vi "ma-resample unevenly sampled input (spline).vi"(0 "X-array in":dbl[](array[numeric]) format="%.2p", 5 "Y-array in":dbl[](array[numeric]) format="%.2p", 7 "dt":dbl=1.0 format="%.2p", 9 "t0":dbl format="%.2p", 11 "error in":errorcluster) -> (4 "X-array out":dbl[](array[numeric]) format="%.2p", 6 "Y-array out":dbl[](array[numeric]) format="%.2p", 8 "evenly sampled waveform out":waveform(dbl), 10 "used t0":dbl format="%.2p", 14 "t0 adjusted warning":bool, 15 "error out":errorcluster)   [LabVIEW 2020, in "NI_MAPro.lvlib"]
doc: "This VI re-samples an unevenly sampled input signal to an evenly sampled waveform according to specified t0 and dt. If the specified t0 value is less than the first value of input X-array (that is the timestamp of the first input sample), then the VI will coerce t0 to the first valid value (greater than X(0)) that also fulfill the relation:\n\nT0_adjusted - t0_in = n * dt_in\n\nThis guarranty that any later comparison of waveforms will be correct with repsect to absolute time."
uses:
  NI_MAPro.lvlib
  NI_AALPro.lvlib
  NI_AALBase.lvlib
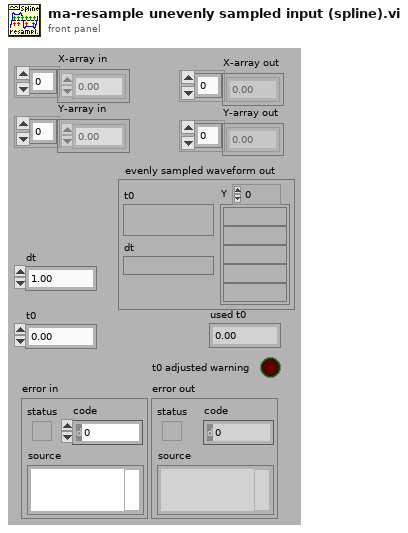
[diagram p1: front panel]
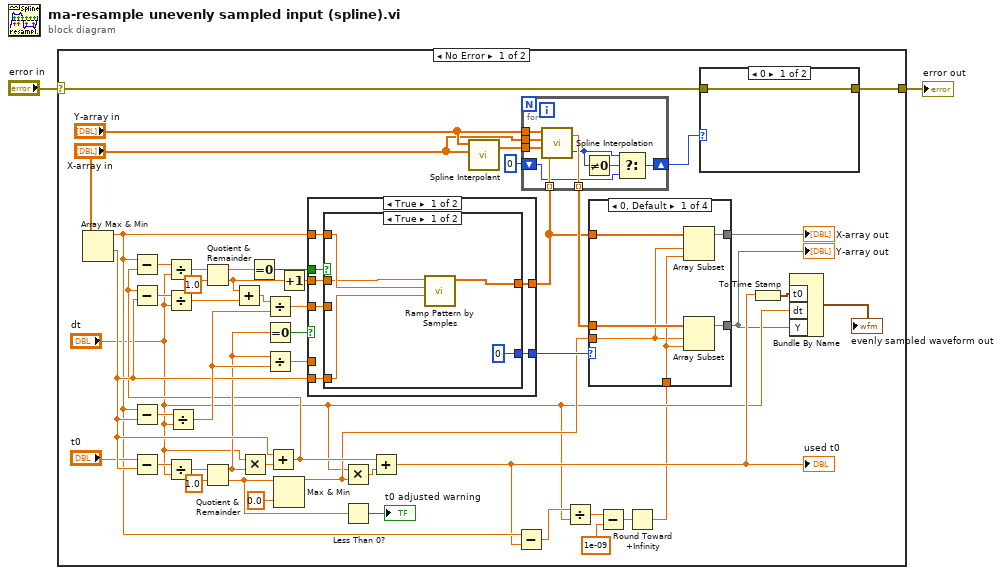
[diagram p0: block diagram]
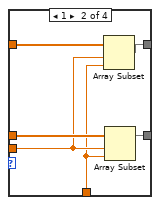
[diagram p2: hidden frame]
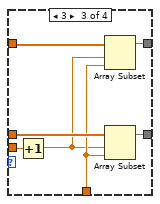
[diagram p3: hidden frame]
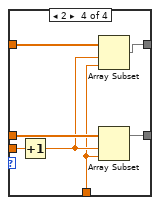
[diagram p4: hidden frame]
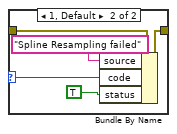
[diagram p5: hidden frame]
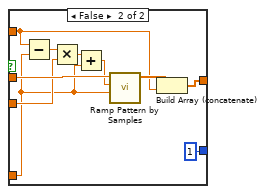
[diagram p6: hidden frame]
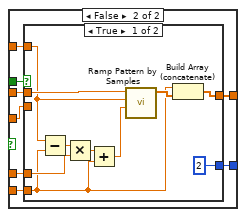
[diagram p7: hidden frame]
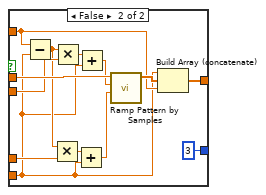
[diagram p8: hidden frame]
diagram:
  n1 = case shown="No Error" "error in" {
    selector: "error in" -> [w24 w147]
    tunnel: [w25 w147] -> w1
    frame No Error {
      n2 = Array Max & Min(array="X-array in") -> (max value=w17:dbl, min value=w31:dbl)  [unwired: 2 out]
      n3 = Subtract(x=w17, y=w31) -> (x-y=w41:dbl)
      n4 = Subtract(x="t0", y=w31) -> (x-y=w33:dbl)
      n5 = Divide(x=w33, y="dt") -> (x/y=w35:dbl)
      n6 = Divide(x=w41, y="dt") -> (x/y=w39:dbl)
      n7 = Quotient & Remainder(x=w35, y=1.0) -> (x-y*floor(x/y)=w30:dbl, floor(x/y)=w23:dbl)
      n8 = Multiply(x="dt", y=w30) -> (x*y=w32:dbl)
      n9 = Equal To 0?(x=w30) -> (x = 0?=w46:bool)
      n10 = Divide(x=w30, y=w39) -> (x/y=w44:dbl)
      n11 = Add(x=w31, y=w32) -> (x+y=w27:dbl)
      n12 = Subtract(x=w17, y=w27) -> (x-y=w50:dbl)
      n13 = Subtract(x=w27, y=w31) -> (x-y=w51:dbl)
      n14 = Divide(x=w50, y="dt") -> (x/y=w40:dbl)
      n15 = Divide(x=w51, y="dt") -> (x/y=w36:dbl)
      n16 = Quotient & Remainder(x=w40, y=1.0) -> (x-y*floor(x/y)=w48:dbl, floor(x/y)=w38:dbl)
      n17 = Add(x=w38, y=w36) -> (x+y=w37:dbl)
      n18 = Equal To 0?(x=w48) -> (x = 0?=w47:bool)
      n19 = Divide(x=w37, y=w39) -> (x/y=w45:dbl)
      n20 = Max & Min(x=w23, y=0.0) -> (max(x,y)=w20:dbl)  [unwired: 1 out]
      n21 = Increment(x=w38) -> (x+1=w42:dbl)
      n22 = case shown="True" w46 {
        tunnel: w47 -> [w91 w114]
        tunnel: w31 -> [w90 w113]
        tunnel: w17 -> [w89 w112]
        tunnel: [w88 w111] -> w18
        tunnel: w42 -> [w87 w110]
        tunnel: w45 -> [w86 w109]
        tunnel: w44 -> [_ w108]
        tunnel: [w85 w107] -> w21
        frame True {
          n23 = case shown="True" w91 {
            tunnel: w90 -> [w96 w98]
            tunnel: w89 -> [w95 w103]
            tunnel: [w94 w105] -> w88
            tunnel: w87 -> [w93 w106]
            tunnel: w86 -> [_ w101]
            tunnel: [0 1] -> w85
            frame True {
              n24 = call "Ramp Pattern by Samples.vi"("start"=w96, "end"=w95, "samples"=w93) -> ("Ramp Pattern"=w94:dbl[])  [unwired: 7 in, 1 out]
            }
            frame False {
              n25 = Subtract(x=w103, y=w98) -> (x-y=w102:dbl)
              n26 = Multiply(x=w102, y=w101) -> (x*y=w99:dbl)
              n27 = Add(x=w99, y=w98) -> (x+y=w100:dbl)
              n28 = call "Ramp Pattern by Samples.vi"("start"=w98, "end"=w100, "samples"=w106) -> ("Ramp Pattern"=w104:dbl[])  [unwired: 7 in, 1 out]
              n29 = Build Array (concatenate)(w104, w103) -> (w105:dbl[])
            }
          }
        }
        frame False {
          n30 = case shown="True" w114 {
            tunnel: w113 -> [w116 w127]
            tunnel: w112 -> [w121 w134]
            tunnel: [w118 w136] -> w111
            tunnel: w110 -> [w124 w137]
            tunnel: w109 -> [_ w133]
            tunnel: w108 -> [w120 w129]
            tunnel: [2 3] -> w107
            frame True {
              n31 = Subtract(x=w121, y=w116) -> (x-y=w123:dbl)
              n32 = Multiply(x=w123, y=w120) -> (x*y=w122:dbl)
              n33 = Add(x=w122, y=w116) -> (x+y=w119:dbl)
              n34 = call "Ramp Pattern by Samples.vi"("start"=w119, "end"=w121, "samples"=w124) -> ("Ramp Pattern"=w117:dbl[])  [unwired: 7 in, 1 out]
              n35 = Build Array (concatenate)(w116, w117) -> (w118:dbl[])
            }
            frame False {
              n36 = Subtract(x=w134, y=w127) -> (x-y=w128:dbl)
              n37 = Multiply(x=w128, y=w129) -> (x*y=w130:dbl)
              n38 = Multiply(x=w128, y=w133) -> (x*y=w131:dbl)
              n39 = Add(x=w130, y=w127) -> (x+y=w126:dbl)
              n40 = Add(x=w131, y=w127) -> (x+y=w132:dbl)
              n41 = call "Ramp Pattern by Samples.vi"("start"=w126, "end"=w132, "samples"=w137) -> ("Ramp Pattern"=w135:dbl[])  [unwired: 7 in, 1 out]
              n42 = Build Array (concatenate)(w127, w135, w134) -> (w136:dbl[])
            }
          }
        }
      }
      n43 = Multiply(x="dt", y=w20) -> (x*y=w29:dbl)
      n44 = Less Than 0?(x=w23) -> (x < 0?=→"t0 adjusted warning":bool)
      n45 = Add(x=w27, y=w29) -> (x+y=w16:dbl)
      "used t0" <- w16
      n46 = call "Spline Interpolant.vi"("X"="X-array in", "Y"="Y-array in") -> ("Interpolant"=w52:dbl[])  [unwired: 2 in, 1 out]
      n47 = Subtract(x=w17, y=w16) -> (x-y=w15:dbl)
      n48 = for {
        tunnel: w52 -> [w146]
        tunnel: "Y-array in" -> [w145]
        tunnel: w18 -> [w144] mode=indexing
        tunnel: [w143] -> w19 mode=indexing
        tunnel: "X-array in" -> [w140]
        shift-right: [w138] -> w4
        shift-left: 0 -> [w139]
        n49 = call "Spline Interpolation.vi"("x value"=w144, "Interpolant"=w146, "X"=w140, "Y"=w145) -> ("error"=w141:i32, "interpolation value"=w143:dbl)
        n50 = Not Equal To 0?(x=w141) -> (x != 0?=w142:bool)
        n51 = Select(t=w141, s=w142, f=w139) -> (s? t:f=w138:i32)
      }
      n52 = Divide(x=w15, y="dt") -> (x/y=w13:dbl)
      n53 = Subtract(x=w13, y=1e-09) -> (x-y=w11:dbl)
      n54 = Round Toward +Infinity(x=w11) -> (ceil(x): smallest int >= x=w10:dbl)
      n55 = case shown="0, Default" w21 {
        tunnel: w19 -> [w56 w63 w68 w77]
        tunnel: [w57 w64 w71 w78] -> w9
        tunnel: w18 -> [w55 w61 w70 w74]
        tunnel: [w58 w62 w69 w75] -> w8
        tunnel: w20 -> [w53 w60 w67 w73]
        tunnel: w10 -> [w54 w59 w66 w72]
        frame 0, Default {
          n56 = Array Subset(array=w55, index=w53, length=w54) -> (w58:dbl[])
          n57 = Array Subset(array=w56, index=w53, length=w54) -> (w57:dbl[])
        }
        frame 1 {
          n58 = Array Subset(array=w61, index=w60, length=w59) -> (w62:dbl[])
          n59 = Array Subset(array=w63, index=w60, length=w59) -> (w64:dbl[])
        }
        frame 3 {
          n60 = Increment(x=w67) -> (x+1=w65:dbl)
          n61 = Array Subset(array=w70, index=w65, length=w66) -> (w69:dbl[])
          n62 = Array Subset(array=w68, index=w65, length=w66) -> (w71:dbl[])
        }
        frame 2 {
          n63 = Increment(x=w73) -> (x+1=w76:dbl)
          n64 = Array Subset(array=w74, index=w76, length=w72) -> (w75:dbl[])
          n65 = Array Subset(array=w77, index=w76, length=w72) -> (w78:dbl[])
        }
      }
      "X-array out" <- w8
      "Y-array out" <- w9
      n66 = case shown="0" w4 {
        selector: w4 -> [_ w82]
        tunnel: w24 -> [w79 w84]
        tunnel: [w79 w83] -> w25
        frame 0 {
        }
        frame 1, Default {
          n67 = Bundle By Name(cluster=w84, "source"="Spline Resampling failed", "code"=w82, "status"=TRUE) -> (w83:errorcluster)
        }
      }
      n68 = To Time Stamp(1:w16) -> (0:w3:timestamp)
      n69 = Bundle By Name("t0"=w3, "dt"="dt", "Y"=w9) -> (→"evenly sampled waveform out":waveform(dbl))  [unwired: 1 in]
    }
    frame Error {
    }
  }
  "error out" <- w1
